vi "Initialize.vi"(0 "VISA resource name":refnum<visa-resource-name>, 5 "ID Query (T: Check)":bool=TRUE, 7 "Reset (T: Reset)":bool=TRUE, 11 "error in (no error)":errorcluster) -> (4 "VISA resource name out":refnum<visa-resource-name>, 15 "error out":errorcluster)   [LabVIEW 2010, in "Stanford Research PS300 Series.lvlib"]
doc: "This VI passes the addressing information in the instrument decriptor to the Instr Open VI and returns the instrument ID. You can optionally reset the instrument by setting the front panel reset control. You must run this VI before using any of the instrument driver VIs for this instrument."
uses:
  <instrlib>/Stanford Research PS300 Series/Stanford Research PS300 Series.lvlib
panel:
  # "© 2005 National Instruments.  ALL RIGHTS RESERVED."
  # "Check\nDon't Check"
  # "Reset\nDon't Reset"
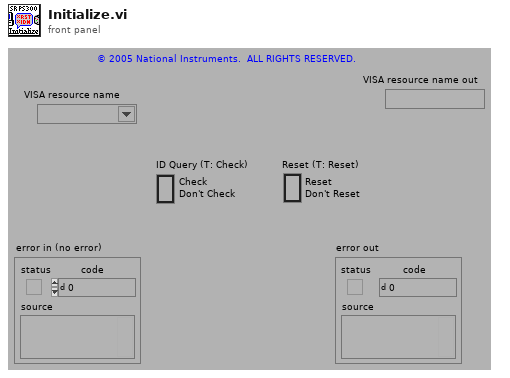
[diagram p1: front panel]
types:
  T1 = cluster{"status":bool, "code":i32, "VI Name":string}
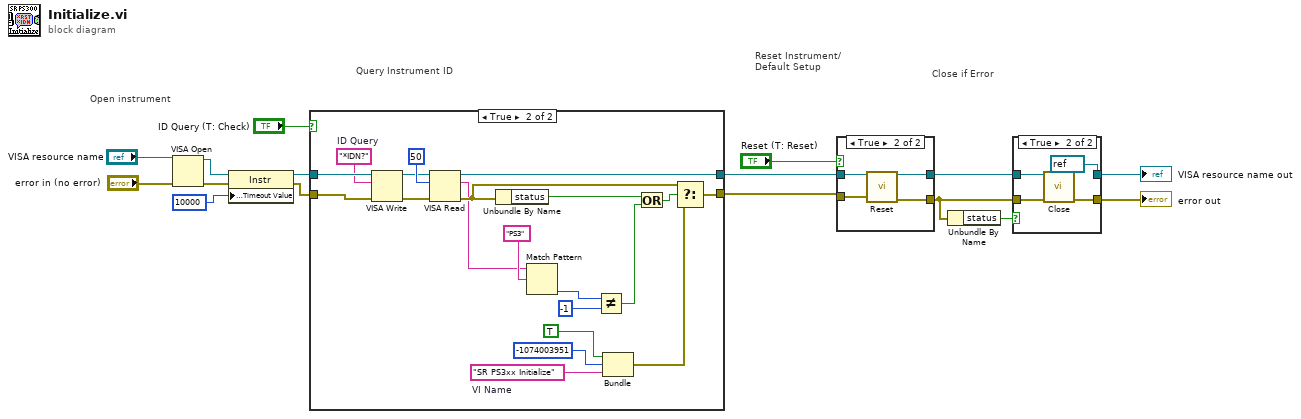
[diagram p0: block diagram]
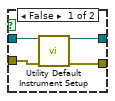
[diagram p3: hidden frame]
diagram:
  # "Close if Error"
  # "Query Instrument ID"
  # "Reset Instrument/\nDefault Setup"
  # "Open instrument"
  n1 = VISA Open(error in (no error)="error in (no error)", VISA resource name="VISA resource name") -> (VISA resource name=w5:refnum<visa-resource-name>, error out=w7:errorcluster)  [unwired: 3 in]
  n2 = property on="Property Node" class="Instr"(reference=w5, error in=w7, "General Settings:Timeout Value"=u32 10000 ("Tmo Value")) -> (reference out=w4:refnum<visa-resource-name>, error out=w6:errorcluster)
  n3 = case shown="True" "ID Query (T: Check)" {
    tunnel: [w17 w38] -> w15
    tunnel: [w18 w35] -> w16
    tunnel: w4 -> [w18 w36]
    tunnel: w6 -> [w17 w37]
    frame False {
    }
    frame True {
      w31 = "*IDN?"  # ID Query
      w21 = "SR PS3xx Initialize"  # VI Name
      n4 = VISA Write(VISA resource name=w36, write buffer=w31, error in (no error)=w37) -> (VISA resource name out=w24:refnum<visa-resource-name>, error out=w26:errorcluster)  [unwired: 1 out]
      n5 = VISA Read(VISA resource name=w24, byte count=u32 50, error in (no error)=w26) -> (VISA resource name out=w35:refnum<visa-resource-name>, read buffer=w23:string, error out=w25:errorcluster)  [unwired: 1 out]
      n6 = Unbundle By Name(w25) -> ("status"=w28:bool)
      n7 = Match Pattern(string=w23, regular expression="PS3") -> (offset past match=w20:i32)  [unwired: 1 in, 3 out]
      n8 = Not Equal?(x=w20, y=-1) -> (x != y?=w22:bool)
      n9 = Bundle(TRUE, -1074003951, "VI Name"=w21) -> (w32:cluster{bool, i32, "VI Name":string})  [unwired: 1 in]
      n10 = Or(x=w28, y=w22) -> (x .or. y?=w27:bool)
      n11 = Select(t=w25, s=w27, f=w32) -> (s? t:f=w38:T1)
    }
  }
  n12 = case shown="True" "Reset (T: Reset)" {
    tunnel: w15 -> [w41 w43]
    tunnel: [w40 w46] -> w10
    tunnel: w16 -> [w42 w44]
    tunnel: [w39 w45] -> w9
    frame False {
      n13 = call <instrlib>:"Utility Default Instrument Setup.vi"("VISA resource name"=w42, "error in (no error)"=w41) -> ("VISA resource name out"=w39:refnum<visa-resource-name>, "error out"=w40:errorcluster)  [unwired: 12 in]
    }
    frame True {
      n14 = call <instrlib>:"Reset.vi"("VISA resource name"=w44, "error in (no error)"=w43) -> ("VISA resource name out"=w45:refnum<visa-resource-name>, "error out"=w46:errorcluster)  [unwired: 12 in]
    }
  }
  n15 = Unbundle By Name(w10) -> ("status"=w11:bool)
  n16 = case shown="True" w11 {
    tunnel: w9 -> [w48 w51]
    tunnel: w10 -> [w47 w52]
    tunnel: [w48 refnum<visa-resource-name> refnum ("VISA resource name out")] -> w3
    tunnel: [w47 w50] -> w2
    frame False {
    }
    frame True {
      n17 = call <instrlib>:"Close.vi"("VISA resource name"=w51, "error in (no error)"=w52) -> ("error out"=w50:errorcluster)  [unwired: 13 in]
    }
  }
  "VISA resource name out" <- w3
  "error out" <- w2
